vi "lv-ros-bridge.vi"(8 "error in (no error)":errorcluster, 9 "Topic string":string="{ \"op\": \"subscribe\", \"topic\" : \"/chatter_joy\" }", 10 "rosbridge port":u16=9090, 11 "rosbridge server IP":string="192.168.5.103") -> (0 "error out":errorcluster, 2 "axes":sgl[](array[numeric]), 3 "buttons":i32[](array[numeric]))   [LabVIEW 2014]
uses:
  <vilib>/Intelligent Energy/WebSockets API/WebSockets/WebSockets.lvlib
panel:
  out "incomming\nmessage":T1
  out "value":T1
  in  "?":T1
  out "raw frame":string
  in  "stop":bool
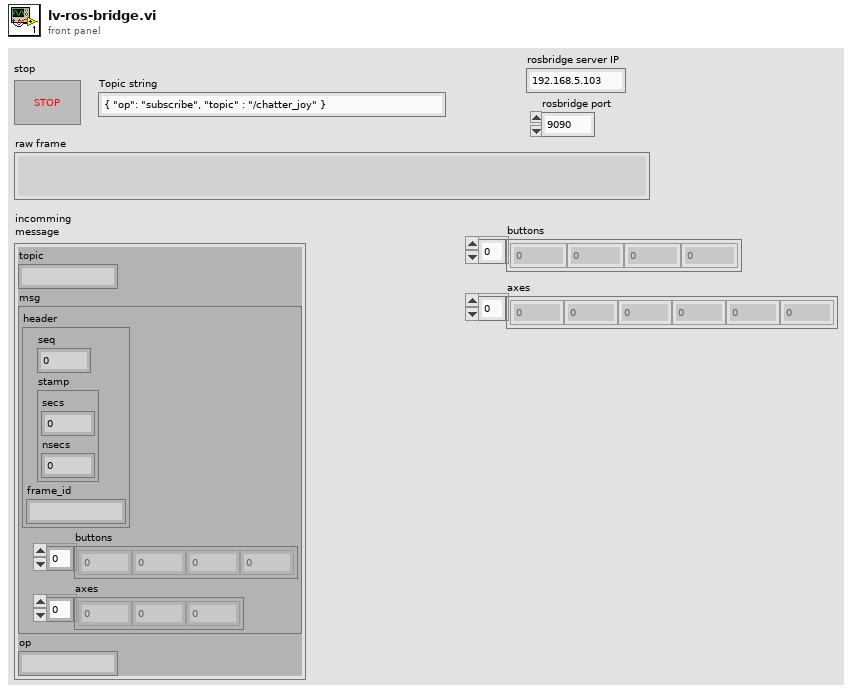
[diagram p1: front panel]
types:
  T1 = cluster{"topic":string, "msg":cluster{"header":cluster{"seq":u32, "stamp":cluster{"secs":u32, "nsecs":i32}, "frame_id":string}, "buttons":i32[], "axes":sgl[]}, "op":string}
  T2 = enum16{"Standard", "Buffered", "CRLF", "Immediate"}
  T3 = cluster{"header":cluster{"seq":u32, "stamp":cluster{"secs":u32, "nsecs":i32}, "frame_id":string}, "buttons":i32[], "axes":sgl[]}
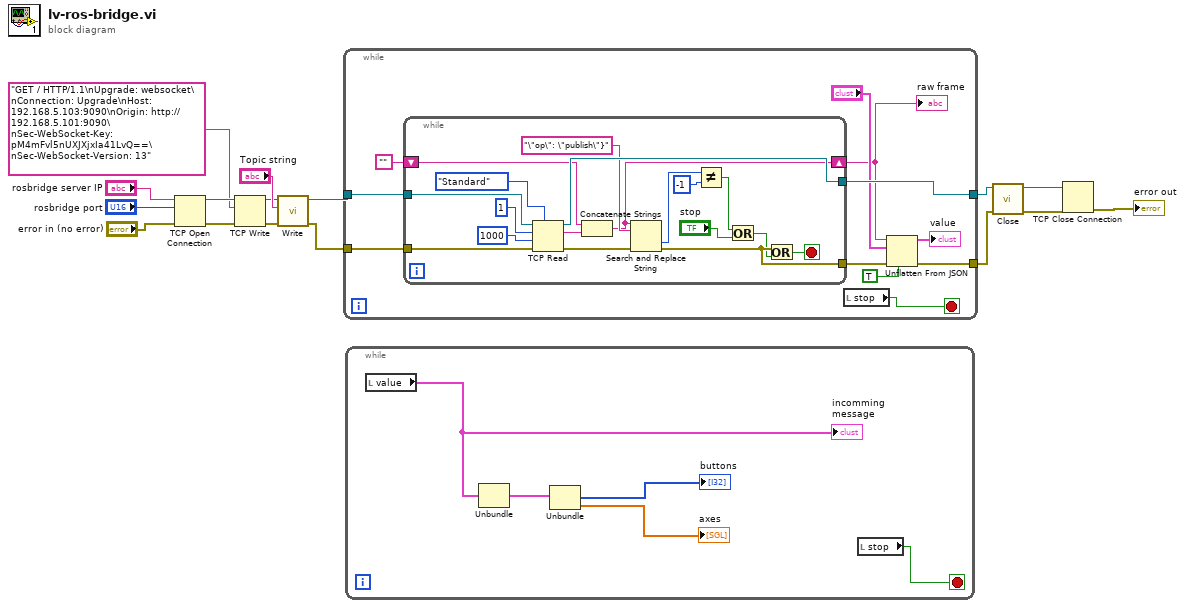
[diagram p0: block diagram]
diagram:
  n1 = TCP Open Connection(address="rosbridge server IP", remote port or service name="rosbridge port", error in (no error)="error in (no error)") -> (connection ID=w14:refnum<k5>, error out=w12:errorcluster)  [unwired: 2 in]
  n2 = TCP Write(connection ID=w14, data in="GET / HTTP/1.1\nUpgrade: websocket\nConnection: Upgrade\nHost: 192.168.5.103:9090\nOrigin: http://192.168.5.101:9090\nSec-WebSocket-Key: pM4mFvl5nUXJXjxIa41LvQ==\nSec-WebSocket-Version: 13", error in (no error)=w12) -> (connection ID out=w8:refnum<k5>, error out=w7:errorcluster)  [unwired: 1 in, 1 out]
  n3 = call <vilib>:"Write.vi"("error in (no error)"=w7, "Data"="Topic string", "WebSocket Connection in"=w8) -> ("error out"=w3:errorcluster, "WebSocket Connection out"=w4:refnum<k5>)  [unwired: 7 in]
  n4 = while {
    tunnel: [w27] -> w6
    tunnel: [w22] -> w5
    tunnel: w4 -> [w26]
    tunnel: w3 -> [w25]
    stop <- w17 stop-if-true
    n5 = while {
      tunnel: [w43] -> w27
      tunnel: [w36] -> w23
      tunnel: w26 -> [w44]
      tunnel: w25 -> [w39]
      shift-right: [w29] -> w20
      shift-left: "" -> [w31]
      stop <- w45 stop-if-true
      n6 = TCP Read(connection ID=w44, bytes to read=1, error in (no error)=w39, 7:T2."Standard" ("mode (standard)"), 9:1000 ("timeout ms (25000)")) -> (connection ID out=w43:refnum<k5>, data out=w30:string, error out=w37:errorcluster)
      n7 = Concatenate Strings(w31, w30) -> (w29:string)
      n8 = Search and Replace String(input string=w29, search string="\"op\": \"publish\"}", error in=w37) -> (offset past replacement=w33:i32, error out=w36:errorcluster)  [unwired: 5 in, 2 out]
      n9 = Not Equal?(x=w33, y=-1) -> (x != y?=w35:bool)
      n10 = Or(x=w35, y="stop") -> (x .or. y?=w32:bool)
      n11 = Or(x=w36, y=w32) -> (x .or. y?=w45:bool)
    }
    "raw frame" <- w20
    n12 = local read "stop"() -> (w17:bool)
    n13 = Unflatten From JSON(JSON string=w20, type and defaults="?", default null elements? (F)=TRUE, error in (no error)=w23) -> (value=→"value":T1, error out=w22:errorcluster)  [unwired: 3 in]
  }
  n14 = while {
    stop <- w46 stop-if-true
    n15 = local read "value"() -> (w50:T1)
    "incomming\nmessage" <- w50
    n16 = Unbundle(w50) -> ("msg"=w49:T3)  [unwired: 2 out]
    n17 = Unbundle(w49) -> ("buttons"=→"buttons":i32[], "axes"=→"axes":sgl[])  [unwired: 1 out]
    n18 = local read "stop"() -> (w46:bool)
  }
  n19 = call <vilib>:"Close.vi"("error in (no error)"=w5, "WebSocket Connection in"=w6) -> ("error out"=w9:errorcluster, "WebSocket Connection in"=w10:refnum<k5>)  [unwired: 8 in]
  n20 = TCP Close Connection(connection ID=w10, error in (no error)=w9) -> (error out=→"error out":errorcluster)  [unwired: 1 in, 1 out]
